vi "test Empty Executable Name.vi"(8 "error in":errorcluster) -> (0 "error out":errorcluster)   [LabVIEW 2024, in "serenial.io-ase.test.lvlib"]
uses:
  serenial.io-ase.test.lvlib
  <vilib>/addons/_JKI Toolkits/Caraya/classes/Assert/Assert.lvclass
  <vilib>/addons/_JKI Toolkits/Caraya/classes/Test/Test.lvclass
  serenial.io-ase/ase/ase.lvclass
  <vilib>/addons/_JKI Toolkits/Caraya/classes/Assert/Assert Equal Value and Type_Variant.vi
  serenial.io-ase/ase/Start Call (Command).vi
  serenial.io-ase/ase/Start Call (Exe-Args).vi
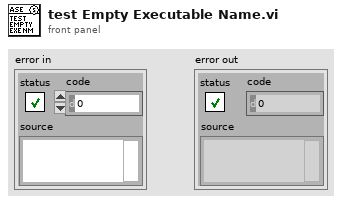
[diagram p1: front panel]
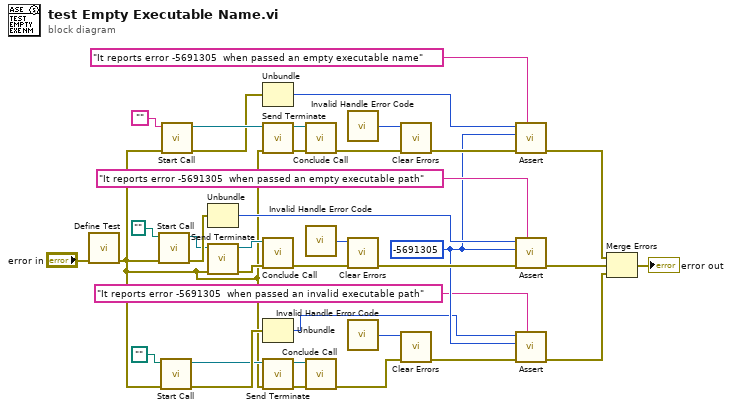
[diagram p0: block diagram]
diagram:
  w3 = -5691305 ("error code (1)")
  n1 = call <vilib>:"Define Test.vi"("error in (no error)"="error in") -> ("error out"=w5:errorcluster)  [unwired: 9 in, 1 out]
  n2 = call-poly "Start Call.vi"("error in"=w5, "Executable Path"=path "") -> ("error out"=w24:errorcluster, "New ASE Handle"=w20:refnum<class "ase.lvclass">)  [unwired: 8 in]
  n3 = call-poly "Start Call.vi"("error in"=w5, "Executable Path"=path "") -> ("error out"=w9:errorcluster, "New ASE Handle"=w6:refnum<class "ase.lvclass">)  [unwired: 8 in]
  n4 = call-poly "Start Call.vi"("error in"=w5, "Command"="") -> ("error out"=w29:errorcluster, "New ASE Handle"=w34:refnum<class "ase.lvclass">)  [unwired: 8 in]
  n5 = Unbundle(w24) -> ("code"=w15:i32)  [unwired: 2 out]
  n6 = call "Send Terminate.vi"("error in"=w5, "ASE Handle"=w20) -> ("error out"=w25:errorcluster, "ASE Handle Duplicate"=w23:refnum<class "ase.lvclass">)  [unwired: 7 in, 1 out]
  n7 = Unbundle(w29) -> ("code"=w35:i32)  [unwired: 2 out]
  n8 = call "Send Terminate.vi"("error in"=w5, "ASE Handle"=w34) -> ("error out"=w28:errorcluster, "ASE Handle Duplicate"=w30:refnum<class "ase.lvclass">)  [unwired: 7 in, 1 out]
  n9 = call "Conclude Call.vi"("error in"=w25, "ASE Handle"=w23) -> ("error out"=w21:errorcluster)  [unwired: 7 in, 2 out]
  n10 = Unbundle(w9) -> ("code"=w2:i32)  [unwired: 2 out]
  n11 = call "Send Terminate.vi"("error in"=w5, "ASE Handle"=w6) -> ("error out"=w8:errorcluster, "ASE Handle Duplicate"=w10:refnum<class "ase.lvclass">)  [unwired: 7 in, 1 out]
  n12 = call "Conclude Call.vi"("error in"=w28, "ASE Handle"=w30) -> ("error out"=w33:errorcluster)  [unwired: 7 in, 2 out]
  n13 = call "Invalid Handle Error Code.vi"() -> ("Invalid Handle Error"=w22:i32)
  n14 = call "Conclude Call.vi"("error in"=w8, "ASE Handle"=w10) -> ("error out"=w12:errorcluster)  [unwired: 7 in, 2 out]
  n15 = call "Invalid Handle Error Code.vi"() -> ("Invalid Handle Error"=w32:i32)
  n16 = call <vilib>:"Clear Errors.vi"("error in (no error)"=w21, "specific error code to clear (0: all)"=w22) -> ("error out"=w18:errorcluster)  [unwired: 4 in, 1 out]
  n17 = call "Invalid Handle Error Code.vi"() -> ("Invalid Handle Error"=w11:i32)
  n18 = call <vilib>:"Clear Errors.vi"("error in (no error)"=w33, "specific error code to clear (0: all)"=w32) -> ("error out"=w31:errorcluster)  [unwired: 4 in, 1 out]
  n19 = call <vilib>:"Clear Errors.vi"("error in (no error)"=w12, "specific error code to clear (0: all)"=w11) -> ("error out"=w13:errorcluster)  [unwired: 4 in, 1 out]
  n20 = call-poly <vilib>:"Assert.vi"("Label"="It reports error -5691305  when passed an empty executable name", "error in (no error)"=w31, "Y"=w3, "X"=w35) -> ("error out"=w27:errorcluster)  [unwired: 6 in, 1 out]
  n21 = call-poly <vilib>:"Assert.vi"("Label"="It reports error -5691305  when passed an empty executable path", "error in (no error)"=w18, "Y"=w3, "X"=w15) -> ("error out"=w16:errorcluster)  [unwired: 6 in, 1 out]
  n22 = call-poly <vilib>:"Assert.vi"("Label"="It reports error -5691305  when passed an invalid executable path", "error in (no error)"=w13, "Y"=w3, "X"=w2) -> ("error out"=w4:errorcluster)  [unwired: 6 in, 1 out]
  n23 = Merge Errors(w27, w16, w4) -> (→"error out":errorcluster)
